vi "RSNRPZ State Checking.vi"(8 "error in (no error)":errorcluster, 10 "State Checking (T: On)":bool=TRUE, 11 "VISA session":refnum<visa-resource-name> caption="VISA resource name") -> (0 "error out":errorcluster, 3 "dup VISA session":refnum<visa-resource-name> caption="VISA resource name")   [LabVIEW 2010]
doc: "This VI switches state checking of the instrument (reading of the Standard Event Register and checking it for error) status subsystem. Driver VIs are using state checking which is by default enabled.\n\nNote:\n\n(1) In debug mode enable state checking.\n\n(2) For better bus throughput and instruments performance disable state checking.\n\n(3) When state checking is disabled driver does not check if correct instrument model or option is used with each of the VIs. This might cause unexpected behaviour of the instrument."
uses:
  rsnrpz_32.dll
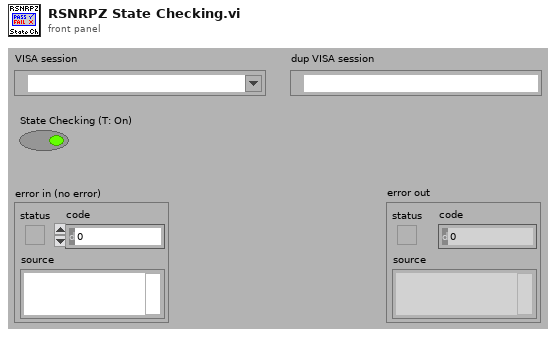
[diagram p1: front panel]
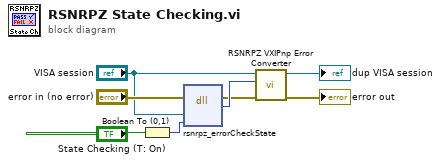
[diagram p0: block diagram]
diagram:
  n1 = Boolean To (0,1)(Boolean="State Checking (T: On)") -> (0, 1=w6:i16)
  n2 = dll-call lib="rsnrpz_32.dll" fn="rsnrpz_errorCheckState"(error in="error in (no error)", "VISA Session"="VISA session", "State Checking"=w6) -> (error out=w5:errorcluster, "Status"=w7:i32)  [unwired: 4 in, 1 out]
  n3 = call <instrlib>:"RSNRPZ VXIPnp Error Converter.vi"("error in"=w5, "VXIPnp error code"=w7, "VISA session"="VISA session") -> ("error out"=→"error out":errorcluster, "dup VISA session"=→"dup VISA session":refnum<visa-resource-name>)  [unwired: 7 in]
